vi "Sans titre 4.vi"   [LabVIEW 2020]
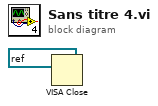
[diagram p0: block diagram]
diagram:
  n1 = VISA Close(VISA resource name=refnum<visa-resource-name> "COM49" ("Nom de ressource VISA")) -> ()  [unwired: 1 in, 1 out]
